vi "Snake.vi"() -> ()   [LabVIEW 2020]
uses:
  Typedef/Snake_states.ctl
panel:
  in  "speed":dbl=700.0 format="%#_13g"
  in  "level":dbl(slide) scale=1.0..5.0
  out "Stop Variable":bool
  out "Score":i32
  out "Snake Field":u32[][](array[colorbox])=[[0, 0, 0, 0, 0, 0, 0, 0, 0, 0, 0, 0, 0, 0, 0, 0, 0, 0, 0, 0, 0, 0, 0, 0, 0, 0, 0], [0, 0, 0, 0, 0, 0, 0, 0, 0, 0, 0, 0, 0, 0, 0, 0, 0, 0, 0, 0, 0, 0, 0, 0, 0, 0, 0], [0, 0, 0, 3622, 0, 0, 0, 0, 0, 0, 0, 0, 0, 0, 0, 0, 0, 0, 0, 0, 0, 0, 0, 0, 0, 0, 0], [0, 0, 0, 0, 0, 0, 0, 0, 0, 0, 0, 0, 0, 0, 0, 0, 0, 0, 0, 0, 0, 0, 0, 0, 0, 0, 0], [0, 0, 0, 0, 0, 0, 0, 0, 0, 0, 0, 0, 0, 0, 0, 0, 0, 0, 0, 0, 0, 0, 0, 0, 0, 0, 0], [0, 0, 0, 0, 0, 0, 0, 0, 0, 0, 0, 0, 0, 0, 0, 0, 0, 0, 0, 0, 0, 0, 0, 0, 0, 0, 0], [0, 0, 0, 0, 0, 0, 0, 0, 0, 0, 0, 0, 0, 0, 0, 0, 0, 0, 0, 0, 0, 0, 0, 0, 0, 0, 0], [0, 0, 0, 0, 0, 0, 0, 0, 0, 0, 0, 0, 0, 0, 0, 0, 0, 0, 0, 0, 0, 0, 0, 0, 0, 0, 0], [0, 0, 0, 0, 0, 0, 0, 0, 0, 0, 0, 0, 0, 0, 0, 0, 0, 0, 0, 0, 0, 0, 0, 0, 0, 0, 0], [0, 0, 0, 0, 0, 0, 0, 0, 0, 0, 0, 0, 0, 0, 0, 0, 0, 0, 0, 0, 0, 0, 0, 0, 0, 0, 0], [0, 0, 0, 0, 0, 0, 0, 0, 0, 0, 0, 0, 0, 0, 0, 0, 0, 0, 0, 0, 0, 0, 0, 0, 0, 0, 0], [0, 0, 0, 0, 0, 0, 0, 0, 0, 0, 0, 0, 0, 0, 0, 0, 0, 0, 0, 0, 0, 0, 0, 0, 0, 0, 0], [0, 0, 0, 0, 0, 0, 0, 0, 0, 0, 0, 0, 0, 0, 0, 0, 0, 0, 0, 0, 0, 0, 0, 0, 0, 0, 0], [0, 0, 0, 0, 0, 0, 0, 0, 0, 0, 0, 0, 0, 0, 0, 0, 0, 0, 0, 0, 0, 0, 0, 0, 0, 0, 0], [0, 0, 0, 0, 0, 0, 0, 0, 0, 0, 0, 0, 0, 0, 0, 0, 0, 0, 0, 0, 0, 0, 0, 0, 0, 0, 0], [0, 0, 0, 0, 0, 0, 0, 0, 0, 0, 0, 0, 0, 0, 0, 0, 0, 0, 0, 0, 0, 0, 0, 0, 0, 0, 0], [0, 0, 0, 0, 0, 0, 0, 0, 0, 0, 0, 0, 0, 0, 0, 0, 0, 0, 0, 0, 0, 0, 0, 0, 0, 0, 0], [0, 0, 0, 0, 0, 0, 0, 0, 0, 0, 0, 0, 0, 0, 0, 0, 0, 0, 0, 0, 0, 0, 0, 0, 0, 0, 0], [0, 0, 0, 0, 0, 0, 0, 0, 0, 0, 0, 0, 0, 0, 0, 0, 0, 0, 0, 0, 0, 0, 0, 0, 0, 0, 0], [0, 0, 0, 0, 0, 0, 0, 0, 0, 0, 0, 0, 0, 0, 0, 0, 0, 0, 0, 0, 0, 0, 0, 0, 0, 0, 0]]
  out "Y Direction":i32
  out "X Direction":i32
  in  "Stop":bool
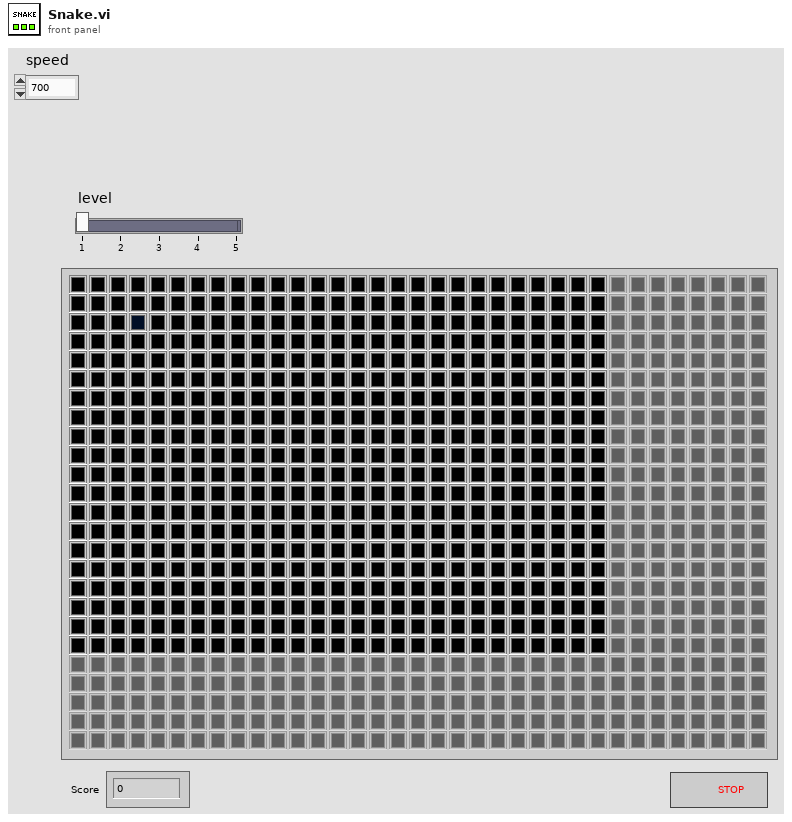
[diagram p1: front panel]
types:
  T1 = typedef "Snake_states.ctl" = enum16{"Initialize", "Start game", "Wait for user to press button", "Stop"}
  T2 = typedef "eventvkey.ctl" = enum16{"ASCII", "Enter", "Return", "Shift", "Ctrl", "Alt", "Cmd", "Opt", "Caps", "NumLock", "Clear", "Break", "Up", "Down", "Left", "Right", "Insert", "Delete", "Home", "End", "PageUp", "PageDown", "Escape", "Help", "Pause", "ScrollLock", "F1", "F2", "F3", "F4", "F5", "F6", "F7", "F8", "F9", "F10", "F11", "F12", "F13", "F14", "F15", "F16", "F17", "F18", "F19", "F20", "F21", "F22", "F23", "F24", "Play", "VolumeUp", "VolumeDown", "Mute", "Two Byte Char"}
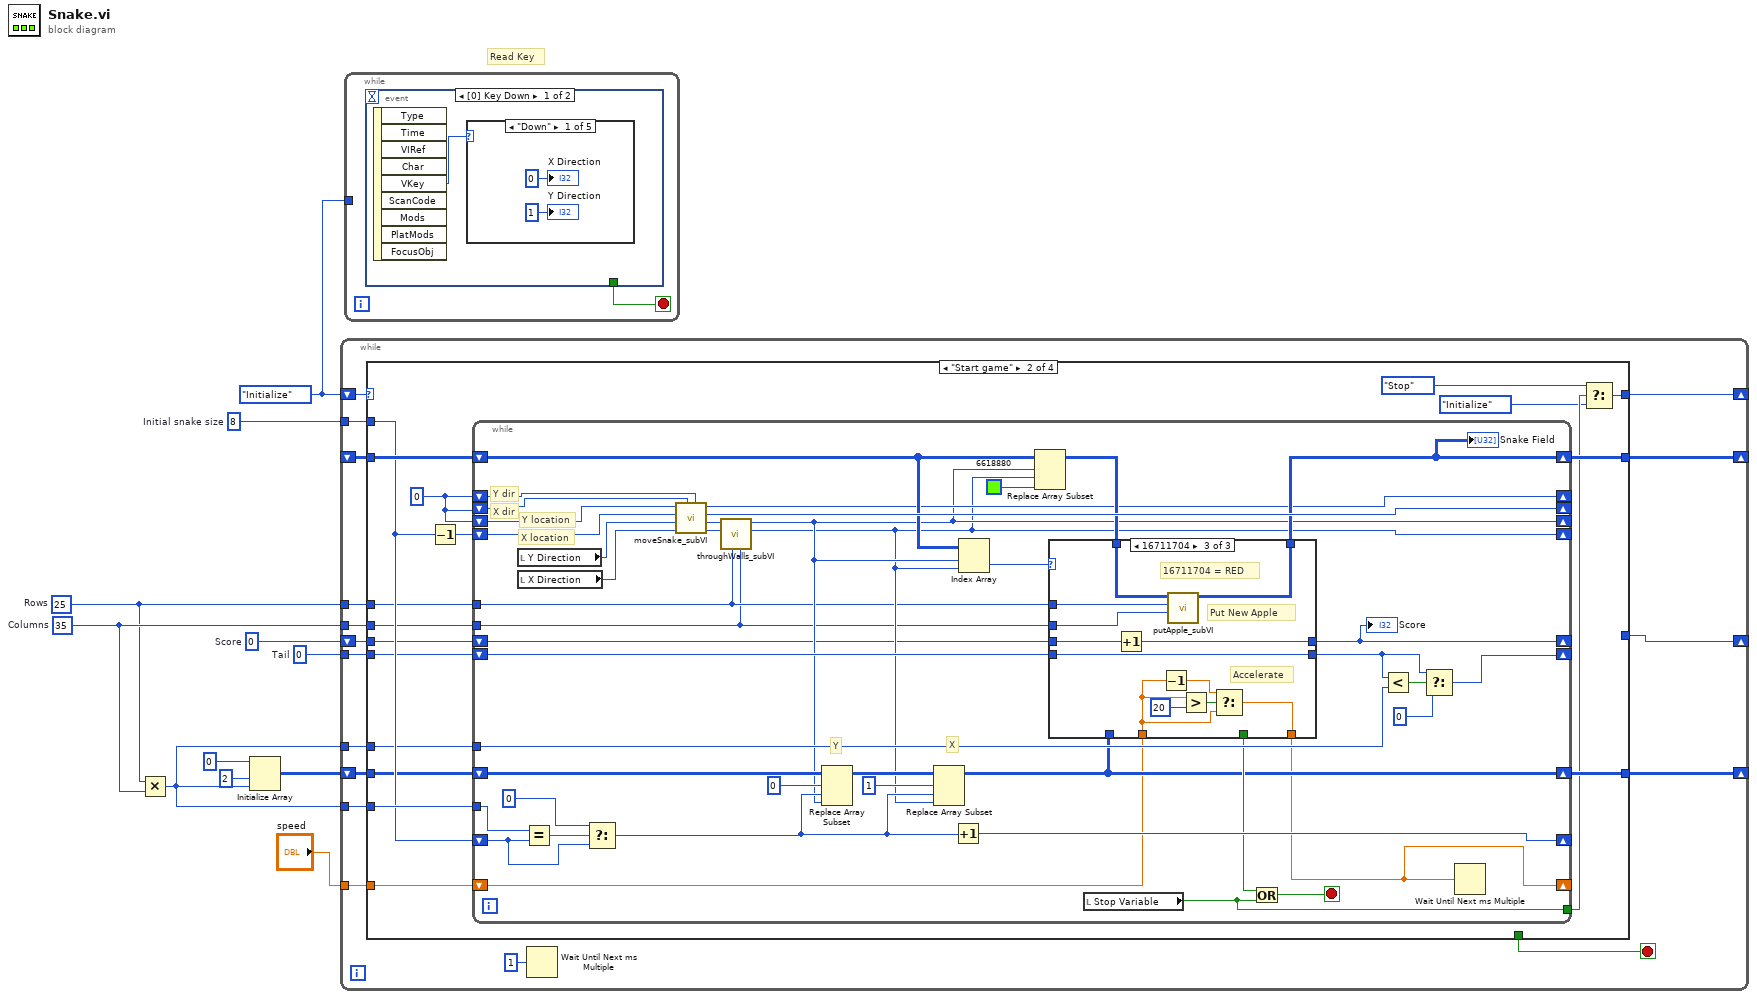
[diagram p0: block diagram]
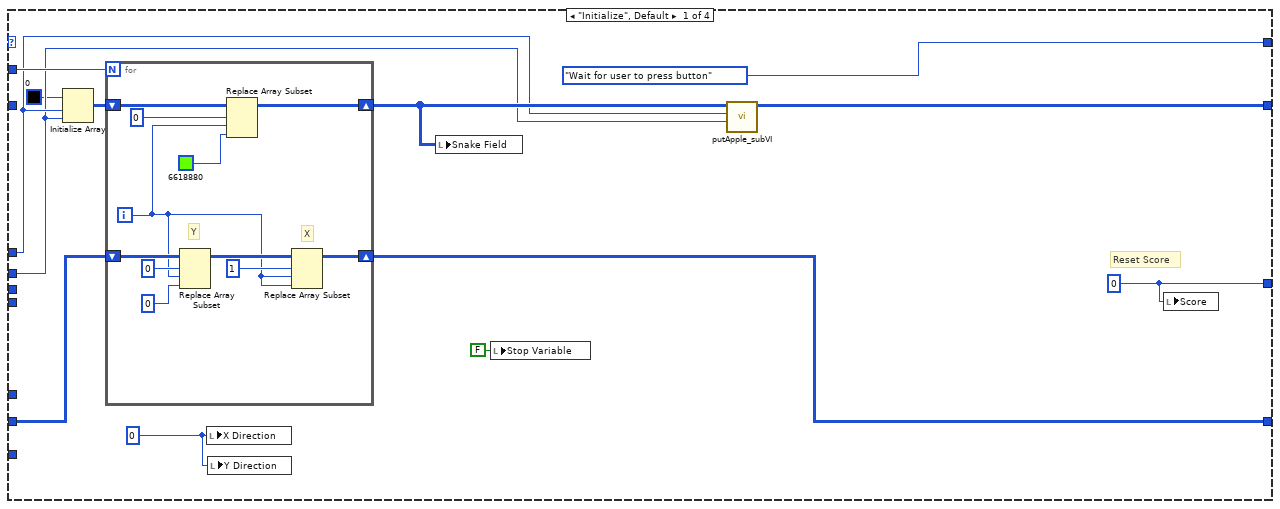
[diagram p2: hidden frame]
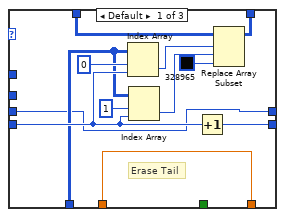
[diagram p3: hidden frame]
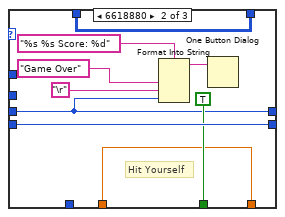
[diagram p4: hidden frame]
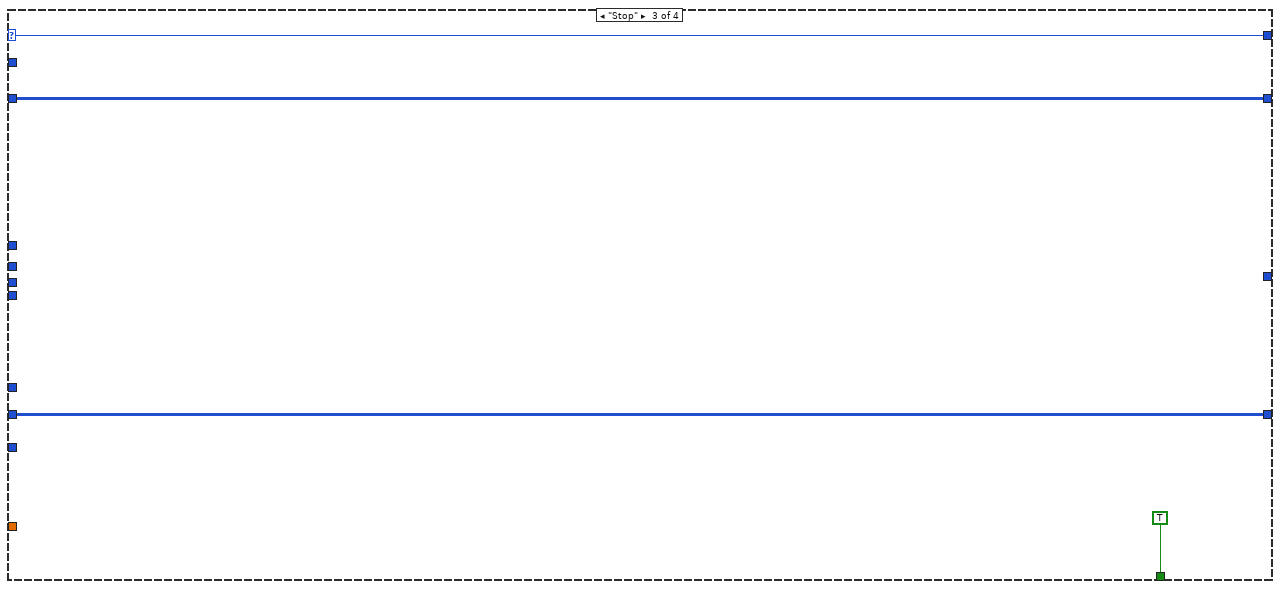
[diagram p5: hidden frame]
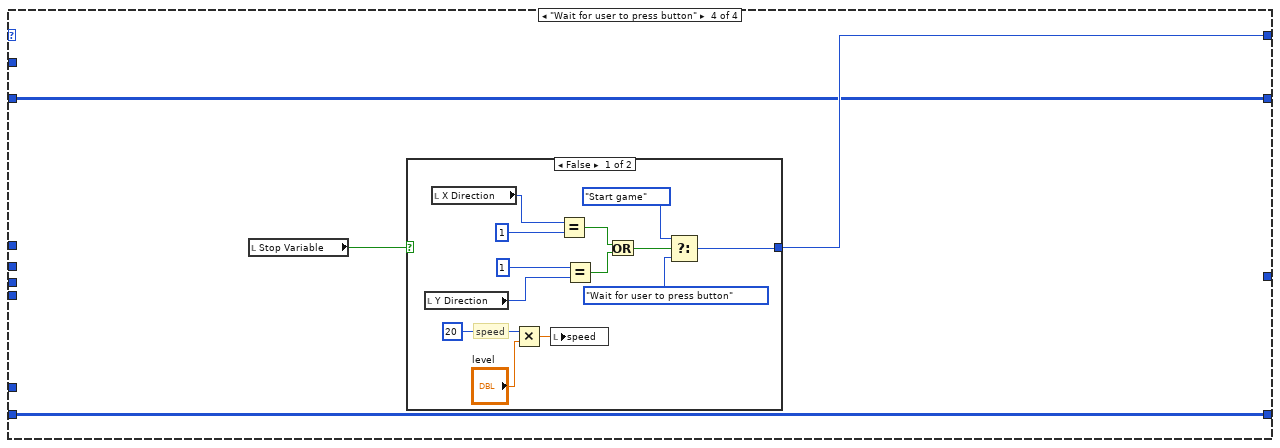
[diagram p6: hidden frame]
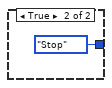
[diagram p7: hidden frame]
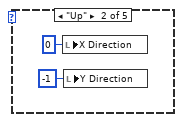
[diagram p8: hidden frame]
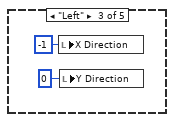
[diagram p9: hidden frame]
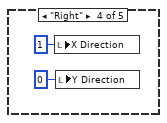
[diagram p10: hidden frame]
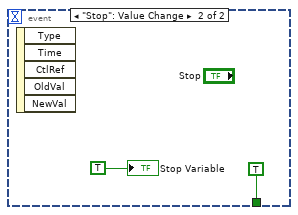
[diagram p12: hidden frame]
diagram:
  w2 = 0  # Score
  w6 = 0  # Tail
  w10 = 8  # Initial snake size
  w5 = 35  # Columns
  w4 = 25  # Rows
  w11 = Snake_states."Initialize"
  # "Read Key"
  n1 = Multiply(x=w4, y=w5) -> (x*y=w3:i32)
  n2 = Initialize Array(0 ("element"), 2 ("dimension size"), w3) -> (w7:i32[][])
  n3 = while {
    shift-right: [w27] -> _
    shift-left: w11 -> [w28]
    tunnel: w3 -> [w25]
    tunnel: w10 -> [w24]
    shift-right: [w23] -> _
    shift-left: _ -> [w26]
    shift-right: [w21] -> _
    shift-left: w7 -> [w22]
    tunnel: w6 -> [w20]
    tunnel: w5 -> [w19]
    tunnel: w4 -> [w18]
    tunnel: w3 -> [w17]
    shift-right: [w14] -> _
    shift-left: w2 -> [w15]
    tunnel: "speed" -> [w13]
    stop <- w16 stop-if-true
    n4 = case shown="\"Start game\"" w28 {
      selector: w28 -> [_ _ w150 _]
      tunnel: [Snake_states."Wait for user to press button" w59 w150 w154] -> w27
      tunnel: w26 -> [_ w70 w149 w153]
      tunnel: w25 -> [_ w69 _ _]
      tunnel: w24 -> [w39 w66 _ _]
      tunnel: [w35 w68 w149 w153] -> w23
      tunnel: w22 -> [w38 w65 w148 w152]
      tunnel: [w37 w64 w148 w152] -> w21
      tunnel: w18 -> [w34 w63 _ _]
      tunnel: w19 -> [w33 w62 _ _]
      tunnel: w20 -> [_ w61 _ _]
      tunnel: w17 -> [_ w60 _ _]
      tunnel: [_ _ TRUE _] -> w16
      tunnel: w15 -> [_ w54 _ _]
      tunnel: [w30 _ _ _] -> w14
      tunnel: w13 -> [_ w53 _ _]
      frame "Initialize", Default {
        w30 = 0 ("index (row)")
        w40 = 0 ("X Direction")
        # "Reset Score"
        n5 = Initialize Array(u32 0 ("Color Box"), w34, w33) -> (w31:u32[][])
        n6 = for {
          N: w39 -> [_]
          shift-right: [w49] -> w36
          shift-left: w31 -> [w51]
          shift-right: [w42] -> w37
          shift-left: w38 -> [w47]
          i -> [w43]
          # "X"
          # "Y"
          n7 = Replace Array Subset(array=w47, new element=0 ("new element/subarray"), index (row)=0, index (col)=w43) -> (w46:i32[][])
          n8 = Replace Array Subset(array=w51, new element=u32 6618880 ("Color Box"), index (row)=0, index (col)=w43) -> (w49:u32[][])
          n9 = Replace Array Subset(array=w46, new element=w43, index (row)=1, index (col)=w43) -> (w42:i32[][])
        }
        n10 = local write "X Direction"(w40) -> ()
        n11 = local write "Y Direction"(w40) -> ()
        n12 = local write "Snake Field"(w36) -> ()
        n13 = local write "Stop Variable"(FALSE ("Stop Variable")) -> ()
        n14 = call "putApple_subVI.vi"("Field Width"=w33, "Field Height"=w34, "Snake Field in"=w36) -> ("Snake Field out"=w35:u32[][])  [unwired: 8 in]
        n15 = local write "Score"(w30) -> ()
      }
      frame "Start game" {
        w55 = 0 ("Current Direction Y")
        n16 = Decrement(x=w66) -> (x-1=w67:i32)
        n17 = while {
          shift-right: [w80] -> _
          shift-left: w55 -> [w113]
          shift-right: [w79] -> _
          shift-left: w67 -> [w112]
          shift-right: [w94] -> w68
          shift-left: w70 -> [w93]
          tunnel: w69 -> [w107]
          shift-right: [w108] -> _
          shift-left: w66 -> [w104]
          shift-right: [w76] -> w64
          shift-left: w65 -> [w103]
          tunnel: w63 -> [w78]
          tunnel: w62 -> [w77]
          shift-right: [w83] -> _
          shift-left: w55 -> [w97]
          shift-right: [w98] -> _
          shift-left: w55 -> [w96]
          shift-right: [w87] -> _
          shift-left: w61 -> [w92]
          tunnel: w60 -> [w91]
          tunnel: [w71] -> w58
          shift-right: [w74] -> _
          shift-left: w54 -> [w75]
          shift-right: [w72] -> _
          shift-left: w53 -> [w73]
          stop <- w85 stop-if-true
          # "X location"
          # "Y location"
          # "X dir"
          # "Y dir"
          # "X"
          # "Y"
          n18 = local read "Y Direction"() -> (w111:i32)
          n19 = local read "X Direction"() -> (w110:i32)
          n20 = Equal?(x=w107, y=w104) -> (x = y?=w106:bool)
          n21 = Select(t=0, s=w106, f=w104) -> (s? t:f=w99:i32)
          n22 = call "moveSnake_subVI.vi"("Old Direction Y"=w97, "Old Direction X"=w96, "New Direction X"=w110, "New Direction Y"=w111, "Snake Head X"=w112, "Snake Head Y"=w113) -> ("New Snake Head X"=w81:i32, "New Snake Head Y"=w82:i32, "Current Direction X"=w98:i32, "Current Direction Y"=w83:i32)  [unwired: 2 in]
          n23 = call "throughWalls_subVI.vi"("Columns"=w77, "Rows"=w78, "Next X"=w81, "Next Y"=w82) -> ("Next X"=w79:i32, "Next Y"=w80:i32)  [unwired: 6 in]
          n24 = Replace Array Subset(array=w103, new element=w80, index (row)=0, index (col)=w99) -> (w102:i32[][])
          n25 = Replace Array Subset(array=w102, new element=w79, index (row)=1, index (col)=w99) -> (w76:i32[][])
          n26 = Increment(x=w99) -> (x+1=w108:i32)
          n27 = Index Array(array=w93, index (row)=w80, index (col)=w79) -> (element=w86:u32)
          n28 = Replace Array Subset(array=w93, new element=u32 6618880 ("Color Box"), index (row)=w80, index (col)=w79) -> (w95:u32[][])
          n29 = case shown="16711704" w86 {
            tunnel: w78 -> [_ _ w145]
            tunnel: w77 -> [_ _ w144]
            tunnel: w95 -> [w125 w134 w146]
            tunnel: [w124 w134 w143] -> w94
            tunnel: w92 -> [w118 w133 w142]
            tunnel: [w117 w133 w142] -> w89
            tunnel: [_ TRUE _] -> w84
            tunnel: w76 -> [w116 _ _]
            tunnel: w75 -> [w115 w128 w141]
            tunnel: [w115 w128 w140] -> w74
            tunnel: w73 -> [w114 w126 w135]
            tunnel: [w114 w126 w136] -> w72
            frame Default {
              # "Erase Tail"
              n30 = Index Array(array=w116, index (row)=0 ("disabled index (row)"), index (col)=w118) -> (element=w119:i32)
              n31 = Index Array(array=w116, index (row)=1, index (col)=w118) -> (element=w122:i32)
              n32 = Increment(x=w118) -> (x+1=w117:i32)
              n33 = Replace Array Subset(array=w125, new element=u32 328965 ("Color Box"), index (row)=w119, index (col)=w122) -> (w124:u32[][])
            }
            frame 6618880 {
              # "Hit Yourself"
              n34 = Format Into String(format string="%s %s Score: %d", "Game Over", "\r", w128) -> (resulting string=w129:string)  [unwired: 2 in, 1 out]
              n35 = One Button Dialog(message=w129) -> ()  [unwired: 1 in, 1 out]
            }
            frame 16711704 {
              # "Accelerate"
              # "16711704 = RED"
              # "Put New Apple"
              n36 = Increment(x=w141) -> (x+1=w140:i32)
              n37 = Decrement(x=w135) -> (x-1=w137:dbl)
              n38 = call "putApple_subVI.vi"("Field Width"=w144, "Field Height"=w145, "Snake Field in"=w146) -> ("Snake Field out"=w143:u32[][])  [unwired: 8 in]
              n39 = Greater?(x=w135, y=u32 20) -> (0:w138:bool)
              n40 = Select(t=w137, s=w138, f=w135) -> (s? t:f=w136:dbl)
            }
          }
          "Snake Field" <- w94
          "Score" <- w74
          n41 = local read "Stop Variable"() -> (w71:bool)
          n42 = Or(x=w84, y=w71) -> (x .or. y?=w85:bool)
          n43 = Less?(x=w89, y=w91) -> (x < y?=w90:bool)
          n44 = Select(t=w89, s=w90, f=0) -> (s? t:f=w87:i32)
          n45 = Wait Until Next ms Multiple(millisecond multiple=w72) -> ()  [unwired: 1 out]
        }
        n46 = Select(t=Snake_states."Stop", s=w58, f=Snake_states."Initialize") -> (s? t:f=w59:T1)
      }
      frame "Stop" {
      }
      frame "Wait for user to press button" {
        n47 = local read "Stop Variable"() -> (w151:bool)
        n48 = case shown="False" w151 {
          tunnel: [w158 Snake_states."Stop"] -> w154
          frame False {
            # "speed"
            n49 = local read "Y Direction"() -> (w167:i32)
            n50 = local read "X Direction"() -> (w165:i32)
            n51 = Multiply(x=u32 20 ("Speed"), y="level") -> (x*y=w157:dbl)
            n52 = local write "speed"(w157) -> ()
            n53 = Equal?(x=w165, y=1) -> (x = y?=w162:bool)
            n54 = Equal?(x=1, y=w167) -> (x = y?=w163:bool)
            n55 = Or(x=w162, y=w163) -> (x .or. y?=w161:bool)
            n56 = Select(t=Snake_states."Start game", s=w161, f=Snake_states."Wait for user to press button") -> (s? t:f=w158:T1)
          }
          frame True {
          }
        }
      }
    }
    n57 = Wait Until Next ms Multiple(millisecond multiple=u32 1) -> ()  [unwired: 1 out]
  }
  n58 = while {
    tunnel: w11 -> [_]
    stop <- w169 stop-if-true
    n59 = event shown="[0] Key Down" {
      selector: _ -> [_ _]
      dyn-events: _ -> [_ _]
      timeout: _ -> [_ _]
      tunnel: [_ TRUE] -> w169
      event Key Down {
        n60 = event-data() -> ("VKey"=w170:T2)  [unwired: 1 in, 8 out]
        n61 = case shown="\"Down\"" w170 {
          frame "Down" {
            "X Direction" <- 0 ("X Direction")
            "Y Direction" <- 1 ("Y Direction")
          }
          frame "Up" {
            n62 = local write "X Direction"(0 ("X Direction")) -> ()
            n63 = local write "Y Direction"(-1 ("Y Direction")) -> ()
          }
          frame "Left" {
            n64 = local write "X Direction"(-1 ("X Direction")) -> ()
            n65 = local write "Y Direction"(0 ("Y Direction")) -> ()
          }
          frame "Right" {
            n66 = local write "X Direction"(1 ("X Direction")) -> ()
            n67 = local write "Y Direction"(0 ("Y Direction")) -> ()
          }
          frame "End", Default {
          }
        }
      }
      event "Stop": Value Change {
        n68 = event-data() -> ()  [unwired: 1 in, 5 out]
        "Stop Variable" <- TRUE
      }
    }
  }
